vi "FPGA informative error on return.vi"(10 "Message":T1, 11 "Class in":refnum<class>) -> (0 "error out":errorcluster)   [LabVIEW 2020]
uses:
  TALOS/TALOS_PPL.lvlibp
  Run Utilities/TypeDefs/Messages/Banana Message.ctl
  Run Utilities/Run Utilities.lvlib
  Run Utilities/TypeDefs/Return Code.ctl
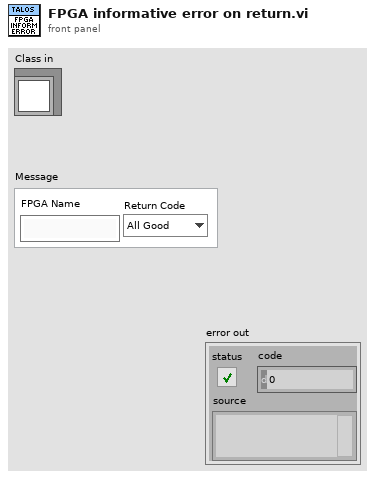
[diagram p1: front panel]
types:
  T1 = typedef "CIRCUS_uServices.lvlib/Run Utilities.lvlib/Banana Message.ctl" = cluster{"FPGA Name":string, "Return Code":T2}
  T2 = typedef "CIRCUS_uServices.lvlib/Run Utilities.lvlib/Return Code.ctl" = enum16{"All Good", "Retry", "Skip", "Skip All", "ABORT"}
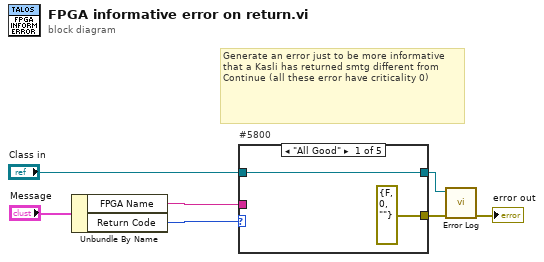
[diagram p0: block diagram]
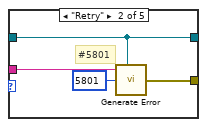
[diagram p2: hidden frame]
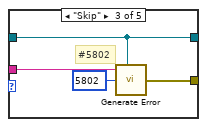
[diagram p3: hidden frame]
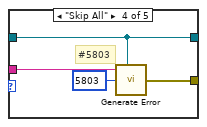
[diagram p4: hidden frame]
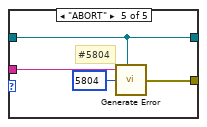
[diagram p5: hidden frame]
diagram:
  # "Generate an error just to be more informative that a Kasli has returned smtg different from Continue (all these error have criticality 0)"
  n1 = Unbundle By Name("Message") -> ("FPGA Name"=w4:string, "Return Code"=w5:T2)
  n2 = case "#5800" shown="\"All Good\"" w5 {
    tunnel: "Class in" -> [w8 w10 w14 w18 w22]
    tunnel: [errorcluster {"status"=FALSE, "code"=0, "source"=""} ("error out") w12 w16 w20 w24] -> w3
    tunnel: w4 -> [_ w11 w15 w19 w23]
    tunnel: [w8 w10 w14 w18 w22] -> w1
    frame "All Good" {
    }
    frame "Retry" {
      # "#5801"
      n3 = call "Generate Error.vi"("Optional String"=w11, "Class"=w10, "Error Code"=5801) -> ("error out"=w12:errorcluster)  [unwired: 4 in]
    }
    frame "Skip" {
      # "#5802"
      n4 = call "Generate Error.vi"("Optional String"=w15, "Class"=w14, "Error Code"=5802) -> ("error out"=w16:errorcluster)  [unwired: 4 in]
    }
    frame "Skip All" {
      # "#5803"
      n5 = call "Generate Error.vi"("Optional String"=w19, "Class"=w18, "Error Code"=5803) -> ("error out"=w20:errorcluster)  [unwired: 4 in]
    }
    frame "ABORT" {
      # "#5804"
      n6 = call "Generate Error.vi"("Optional String"=w23, "Class"=w22, "Error Code"=5804) -> ("error out"=w24:errorcluster)  [unwired: 4 in]
    }
  }
  n7 = call "Error Log.vi"("error in (no error)"=w3, "Object in"=w1) -> ("error out"=→"error out":errorcluster)  [unwired: 9 in]
